vi "Strip path.vi"(3 "Path":string) -> (0 "Name":string, 1 "Stripped path":string)   [LabVIEW 2016, in "RT Management.lvlib" / "File Transfer Behavior.lvclass"]
doc: "Returns the \"Name\" of the last component of a path and the \"Stripped path\" that leads to that component. This VI handles the formatting of the paths, so that they are always returned as valid paths."
uses:
  File Transfer Behavior.lvclass
  Fix path [scalar].vi
  <vilib>/Utility/error.llb/Trim Whitespace.vi
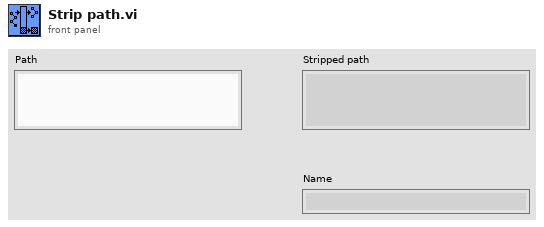
[diagram p1: front panel]
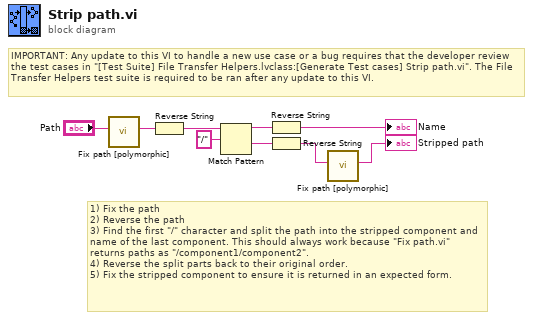
[diagram p0: block diagram]
diagram:
  # "1) Fix the path\n2) Reverse the path\n3) Find the first \"/\" character and split the path into the stripped component and name of the last component. This should always work because \"Fix path.vi\" returns paths as \"/component1/component2\".\n4) Reverse the split parts back to their original order.\n5) Fix the stripped component to ensure it is returned in an expected form."
  # "IMPORTANT: Any update to this VI to handle a new use case or a bug requires that the developer review the test cases in \"[Test Suite] File Transfer Helpers.lvclass:[Generate Test cases] Strip path.vi\". The File Transfer Helpers test suite is required to be ran after any update to this VI."
  n1 = call-poly "Fix path [polymorphic].vi"("Path in"="Path") -> ("Path out"=w5:string)  [unwired: 8 in, 2 out]
  n2 = Reverse String(1:w5) -> (0:w1:string)
  n3 = Match Pattern(string=w1, regular expression="/") -> (before substring=w8:string, after substring=w9:string)  [unwired: 1 in, 2 out]
  n4 = Reverse String(1:w8) -> (0:→"Name":string)
  n5 = Reverse String(1:w9) -> (0:w4:string)
  n6 = call-poly "Fix path [polymorphic].vi"("Path in"=w4) -> ("Path out"=→"Stripped path":string)  [unwired: 8 in, 2 out]
